vi "Write value.vi"(8 "error in (no error)":errorcluster, 10 "value (NULL)":variant, 11 "id in":refnum<class "id.lvclass">) -> (0 "error out":errorcluster, 3 "id out":refnum<class "id.lvclass">)   [LabVIEW 2015]
uses:
  <vilib>/Utility/Data Type/NI_Data Type.lvlib
  <vilib>/Utility/Data Type/Type Definitions/Data Type.ctl
  id.lvclass
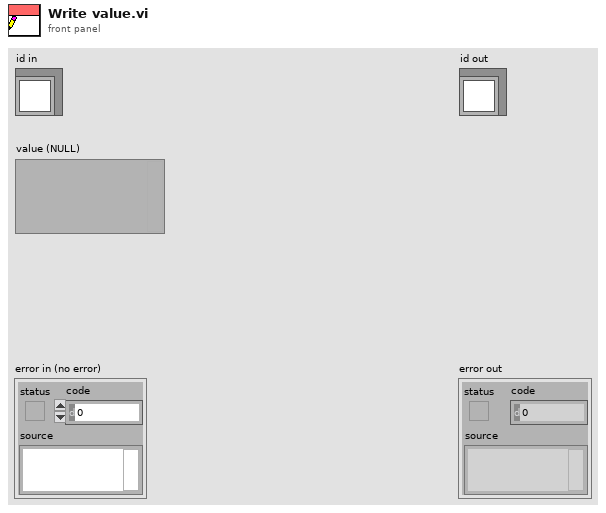
[diagram p1: front panel]
types:
  T1 = typedef "NI_Data Type.lvlib/Data Type.ctl" = enum8{"Invalid Type", "Void", "I8", "I16", "I32", "I64", "U8", "U16", "U32", "U64", "Single Float", "Double Float", "Extended Float", "Single Complex", "Double Complex", "Extended Complex", "Enum U8", "Enum U16", "Enum U32", "Enum U64", "Single Float With Unit", "Double Float With Unit", "Extended Float With Unit", "Single Complex with Unit", "Double Complex with Unit", "Extended Complex with Unit", "Boolean", "String", "Path", "Picture", "Tag", "Array", "Cluster", "Variant", "LV Variant", "Waveform", "Timestamp", "Digital Waveform", "Digital Data", "ExpressData", "Refnum", "External Data", "VI", "Poly VI", "LabVIEW Class Instance", "Fixed Point"}
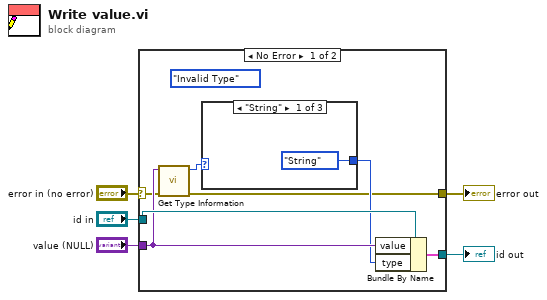
[diagram p0: block diagram]
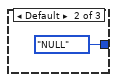
[diagram p2: hidden frame]
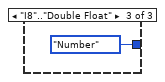
[diagram p3: hidden frame]
diagram:
  n1 = case shown="No Error" "error in (no error)" {
    selector: "error in (no error)" -> [w7 w16]
    tunnel: [w6 w16] -> w4
    tunnel: [w11 w17] -> w2
    tunnel: "id in" -> [w12 w17]
    tunnel: "value (NULL)" -> [w10 _]
    frame No Error {
      (unwired) Data_Type."Invalid Type" ("Type")
      n2 = call <vilib>:"Get Type Information.vi"("error in (no error)"=w7, "Variant"=w10) -> ("error out"=w6:errorcluster, "Type"=w9:T1)  [unwired: 5 in, 3 out]
      n3 = case shown="\"String\"" w9 {
        tunnel: [enum16{"none", "String", "Number", "NULL"}."String" ("type") enum16{"none", "String", "Number", "NULL"}."NULL" ("type") enum16{"none", "String", "Number", "NULL"}."Number" ("type")] -> w8
        frame "String" {
        }
        frame Default {
        }
        frame "I8".."Double Float" {
        }
      }
      n4 = Bundle By Name(cluster=w12, "value"=w10, "type"=w8) -> (w11:cluster{})
    }
    frame Error {
    }
  }
  "error out" <- w4
  "id out" <- w2
